vi "actuator-output-main.vi"   [LabVIEW 2017]
uses:
  <vilib>/Rock Robotics/WPI/Solenoid/WPI_SolenoidSetEnum.vi
types:
  T1 = typedef "WPI_SolenoidDevRef.ctl" = cluster{"DevStatus":errorcluster, "Pneumatics Control Module":u8, "Forward Solenoid Channel":T2, "Reverse Solenoid Channel":T2}
  T2 = typedef "WPI_SolenoidChannel.ctl" = enum8{"Solenoid 0", "Solenoid 1", "Solenoid 2", "Solenoid 3", "Solenoid 4", "Solenoid 5", "Solenoid 6", "Solenoid 7", "Invalid"}
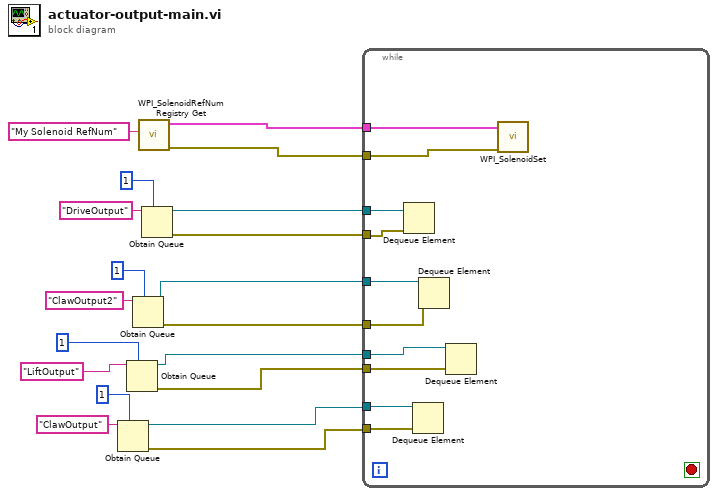
[diagram p0: block diagram]
diagram:
  n1 = Obtain Queue(max queue size (-1, unlimited)=1, name (unnamed)="ClawOutput") -> (queue out=w11:refnum<queue>, error out=w12:errorcluster)  [unwired: 3 in, 1 out]
  n2 = Obtain Queue(max queue size (-1, unlimited)=1, name (unnamed)="LiftOutput") -> (queue out=w13:refnum<queue>, error out=w14:errorcluster)  [unwired: 3 in, 1 out]
  n3 = Obtain Queue(max queue size (-1, unlimited)=1, name (unnamed)="ClawOutput2") -> (queue out=w9:refnum<queue>, error out=w10:errorcluster)  [unwired: 3 in, 1 out]
  n4 = call <vilib>:"WPI_SolenoidRefNum Registry Get.vi"("refnum name"="My Solenoid RefNum") -> ("error out"=w2:errorcluster, "SolenoidDevRef"=w1:T1)  [unwired: 9 in]
  n5 = Obtain Queue(max queue size (-1, unlimited)=1, name (unnamed)="DriveOutput") -> (queue out=w3:refnum<queue>, error out=w4:errorcluster)  [unwired: 3 in, 1 out]
  n6 = while {
    tunnel: w1 -> [w29]
    tunnel: w2 -> [w28]
    tunnel: w3 -> [w27]
    tunnel: w4 -> [w26]
    tunnel: w9 -> [w25]
    tunnel: w10 -> [w24]
    tunnel: w11 -> [w23]
    tunnel: w12 -> [w22]
    tunnel: w13 -> [w21]
    tunnel: w14 -> [w20]
    stop <- _ stop-if-true
    n7 = Dequeue Element(queue=w27, error in (no error)=w26) -> ()  [unwired: 1 in, 4 out]
    n8 = Dequeue Element(queue=w23, error in (no error)=w22) -> ()  [unwired: 1 in, 4 out]
    n9 = Dequeue Element(queue=w25, error in (no error)=w24) -> ()  [unwired: 1 in, 4 out]
    n10 = Dequeue Element(queue=w21, error in (no error)=w20) -> ()  [unwired: 1 in, 4 out]
    n11 = call-poly <vilib>:"WPI_SolenoidSet.vi"("error in (no error)"=w28, "SolenoidDevRef"=w29) -> ()  [unwired: 8 in, 2 out]
  }
